vi "parseErrorCheck.vi"(2 "type":string="bool", 3 "error in":errorcluster) -> (0 "error out":errorcluster)   [LabVIEW 2012]
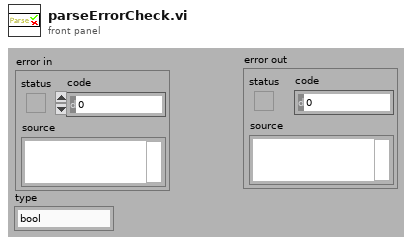
[diagram p1: front panel]
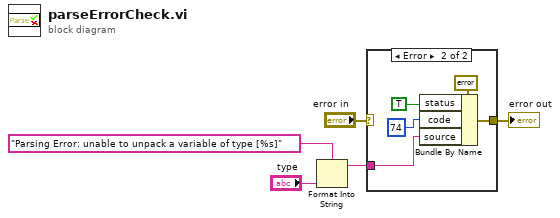
[diagram p0: block diagram]
diagram:
  n1 = Format Into String(format string="Parsing Error: unable to unpack a variable of type [%s]", "type") -> (resulting string=w1:string)  [unwired: 2 in, 1 out]
  n2 = case shown="Error" "error in" {
    selector: "error in" -> [w6 _]
    tunnel: [w6 w11] -> w4
    tunnel: w1 -> [_ w7]
    frame No Error {
    }
    frame Error {
      n3 = Bundle By Name(cluster=errorcluster {"status"=FALSE, "code"=0, "source"=""} ("error IO"), "status"=TRUE, "code"=74, "source"=w7) -> (w11:errorcluster)
    }
  }
  "error out" <- w4
